vi "VIPM_Load File Group Paths.vi"(8 "error in (no error)":errorcluster, 10 "File Group Name":string, 11 "Refnum in":T1) -> (0 "error out":errorcluster, 2 "File Group Paths":string[](array[string]), 3 "Refnum out":T1)   [LabVIEW 2019, in "Project.Dependencies Finder.lvlib" / "Dependency Source_VIPM.lvclass"]
doc: "Load all vi, llb, vims, ctl and lvclass paths from a File Group.s"
uses:
  Dependency Source_VIPM.lvclass
  <vilib>/Utility/config.llb/Config Data RefNum.ctl
  <vilib>/Utility/config.llb/NI_LVConfig.lvlib
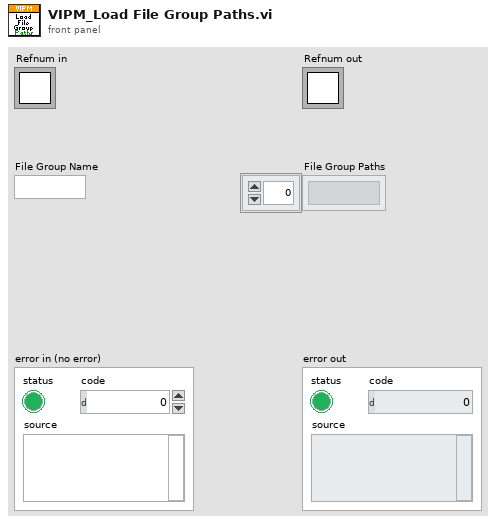
[diagram p1: front panel]
types:
  T1 = typedef "NI_LVConfig.lvlib/Config Data RefNum.ctl" = refnum<k1>
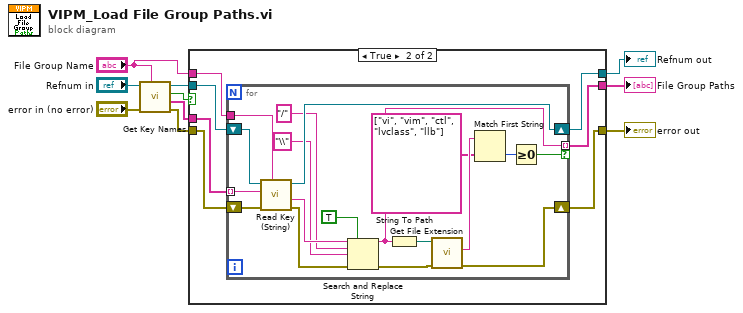
[diagram p0: block diagram]
diagram:
  n1 = call <vilib>:"Get Key Names.vi"("section"="File Group Name", "error in (no error)"="error in (no error)", "refnum"="Refnum in") -> ("error out"=w8:errorcluster, "key names"=w9:string[], "section exists?"=w4:bool, "refnum out"=w6:T1)  [unwired: 5 in]
  n2 = case shown="True" w4 {
    tunnel: [w12 w14] -> w5
    tunnel: w6 -> [w12 w19]
    tunnel: [w11 w15] -> w7
    tunnel: w8 -> [w11 w16]
    tunnel: w9 -> [_ w18]
    tunnel: "File Group Name" -> [_ w17]
    tunnel: [_ w13] -> w1
    frame False {
    }
    frame True {
      n3 = for {
        tunnel: w18 -> [w36] mode=indexing
        tunnel: w17 -> [w35]
        shift-right: [w34] -> w14
        shift-left: w19 -> [w37]
        shift-right: [w28] -> w15
        shift-left: w16 -> [w33]
        tunnel: [w21] -> w13 mode=indexing if=w20
        n4 = call <vilib>:"Read Key (String).vi"("section"=w35, "error in (no error)"=w33, "key"=w36, "refnum"=w37) -> ("error out"=w32:errorcluster, "value"=w25:string, "refnum out"=w34:T1)  [unwired: 4 in, 1 out]
        n5 = Search and Replace String(replace all?=TRUE ("replace all? (F)"), input string=w25, search string="/", replace string="\\" ("search string"), error in=w32) -> (result string=w21:string, error out=w26:errorcluster)  [unwired: 3 in, 2 out]
        n6 = String To Path(string=w21) -> (path=w27:path)
        n7 = call <vilib>:"Get File Extension.vi"("error in (no error)"=w26, "file"=w27) -> ("error out"=w28:errorcluster, "lowercase file extension"=w30:string)  [unwired: 5 in, 3 out]
        n8 = Match First String(2:string[] ["vi", "vim", "ctl", "lvclass", "llb"] ("string array"), 3:w30) -> (0:w31:i32)  [unwired: 1 out]
        n9 = Greater Or Equal To 0?(x=w31) -> (x >= 0?=w20:bool)
      }
    }
  }
  "error out" <- w7
  "Refnum out" <- w5
  "File Group Paths" <- w1
